vi "SetListParameter.vi"() -> ()   [LabVIEW 2018, in "BK Precision 983X Series.lvlib"]
doc: "Set a list parameter value. The complete set should be set and then the \"list save\" command will add the list element to the complete list."
uses:
  <instrlib>/BK Precision 983X Series/BK Precision 983X Series.lvlib
panel:
  in  "Value":dbl
  out "Command":string
  in  "Parameter":T1(ring)
  in  "error in (no error)":errorcluster
  in  "VISA resource name":refnum<visa-resource-name>
  out "error out":errorcluster
  out "VISA resource name out":refnum<visa-resource-name>
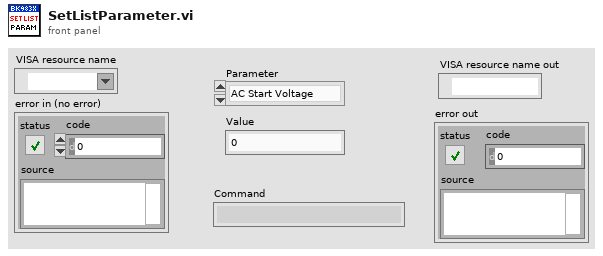
[diagram p1: front panel]
types:
  T1 = enum16{"AC Start Voltage", "AC End Voltage", "DC Start Voltage", "DC End Voltage", "Frequency Start", "Frequency End", "Number of steps (stepno)"}
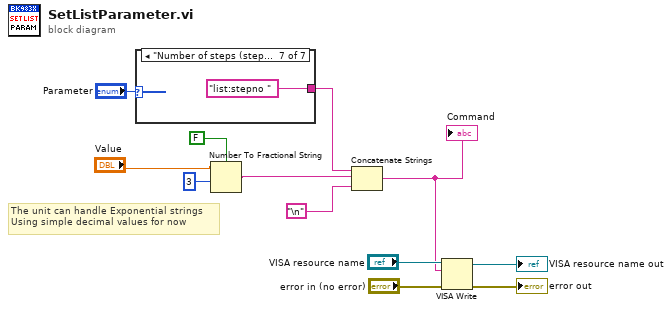
[diagram p0: block diagram]
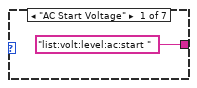
[diagram p2: hidden frame]
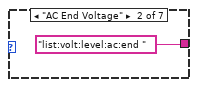
[diagram p3: hidden frame]
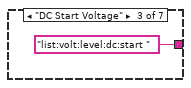
[diagram p4: hidden frame]
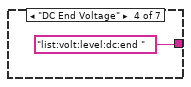
[diagram p5: hidden frame]
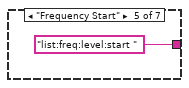
[diagram p6: hidden frame]
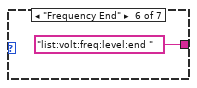
[diagram p7: hidden frame]
diagram:
  # "The unit can handle Exponential strings\nUsing simple decimal values for now"
  n1 = case shown="\"Number of steps (stepno)\"" "Parameter" {
    tunnel: ["list:volt:level:ac:start " "list:volt:level:ac:end " "list:volt:level:dc:start " "list:volt:level:dc:end " "list:freq:level:start " "list:volt:freq:level:end " "list:stepno "] -> w8
    frame "AC Start Voltage" {
    }
    frame "AC End Voltage" {
    }
    frame "DC Start Voltage" {
    }
    frame "DC End Voltage" {
    }
    frame "Frequency Start" {
    }
    frame "Frequency End" {
    }
    frame "Number of steps (stepno)" {
    }
  }
  n2 = Number To Fractional String(use system decimal point (T)=FALSE, number="Value", precision (6)=i16 3) -> (F-format string=w4:string)  [unwired: 1 in]
  n3 = Concatenate Strings(w8, w4, "\n") -> (w10:string)
  "Command" <- w10
  n4 = VISA Write(VISA resource name="VISA resource name", write buffer=w10, error in (no error)="error in (no error)") -> (VISA resource name out=→"VISA resource name out":refnum<visa-resource-name>, error out=→"error out":errorcluster)  [unwired: 1 out]
